vi "dmm_loop_copy_paste_array.vi"(10 "UUT single-ended scan array ref":refnum<vi>, 11 "Copypaste commloop ref":refnum<vi>) -> ()   [LabVIEW 2012]
panel:
  in  "Protocol definition":T1(array[cluster]) {"Variables" items=["Undefined", "Density", "Delta to", "DZDT DeltaT", "Drive mA", "Board Temp", "Mass Flow", "Tube Frequency", "LPO Amp (Filt)", "RPO Amp (Filt)", "LPO Amp (Pk Det)", "RPO Amp (Pk Det)", "Mass Total", "CP Input Volts", "Temp Line", "Drive Gain%", "Flow cal factor", "Status Word 1", "Status Word 2", "Status Word 3", "Status Word 4", "Status Word 5", "Status Word 6"]; "Protocols" items=["None", "MODBUS", "HART", "Fieldbus", "Profibus DP", "Profibus PA"]}
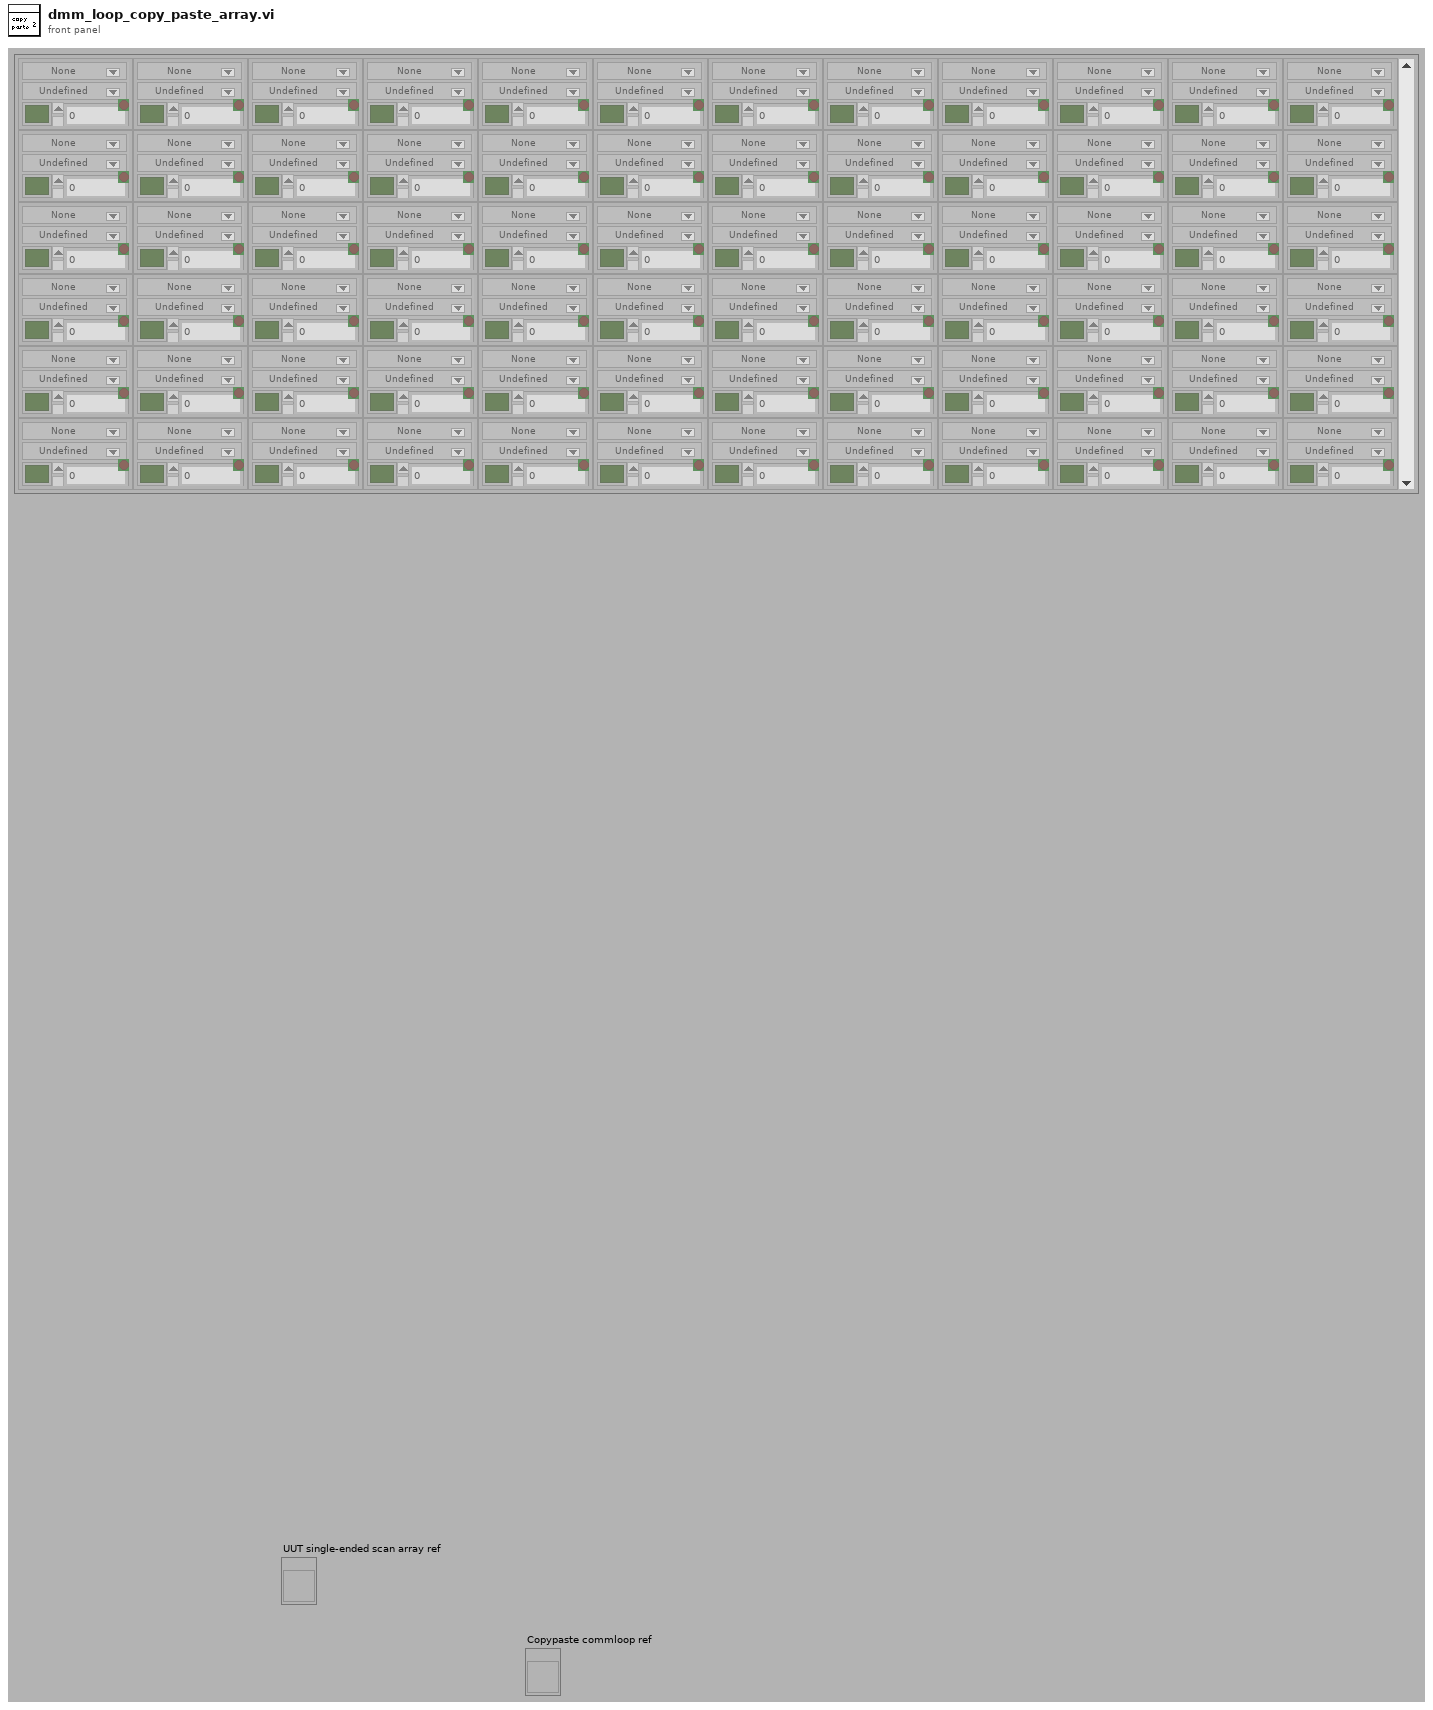
[diagram p1: front panel]
types:
  T1 = cluster{"Protocols":u16, "Variables":u16, "Value":dbl, "Enabled":bool, "Error":bool}[][]
  T2 = cluster{"on?":bool, "Label":string, "measurement type":enum16{"Voltage", "Frequency", "Resistance"}, "Numeric 2":dbl, "current time":timestamp}[][]
  T3 = cluster{"on?":bool, "Label":string, "measurement type":enum16{"Voltage", "Frequency"}, "Numeric 2":dbl, "current time":timestamp}
  T4 = cluster{"on?":bool, "Label":string, "measurement type":enum16{"Voltage", "Frequency", "Resistance"}, "Numeric 2":dbl, "current time":timestamp}[]
  T5 = cluster{"on?":bool, "Label":string, "measurement type":enum16{"Voltage", "Frequency"}, "Numeric 2":dbl, "current time":timestamp}[]
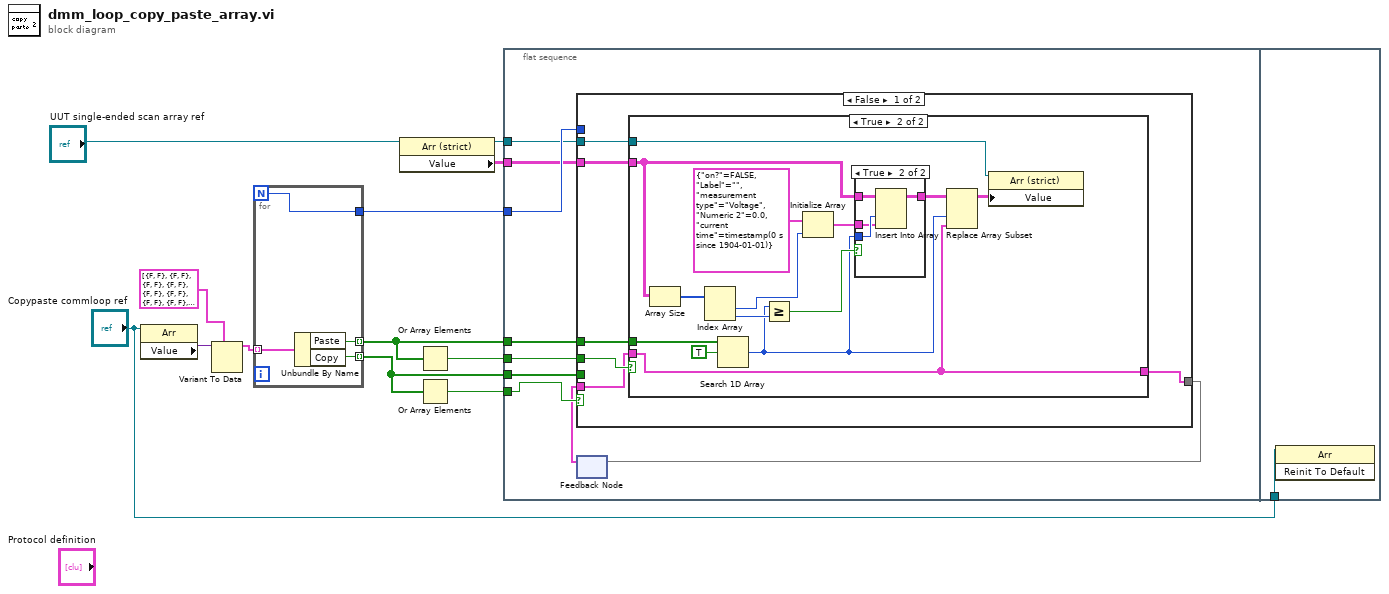
[diagram p0: block diagram]
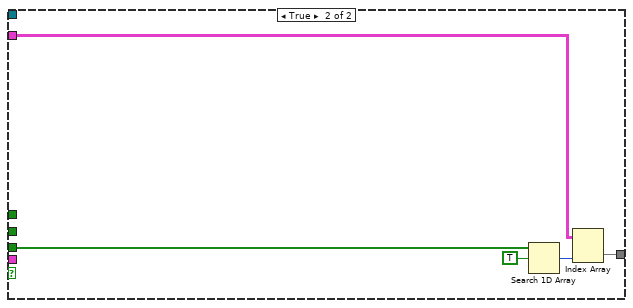
[diagram p4: hidden frame]
diagram:
  n1 = property class="Arr"(reference="Copypaste commloop ref") -> ("Value"=w6:variant)  [unwired: 1 in, 2 out]
  n2 = Variant To Data(type=cluster{"Copy":bool, "Paste":bool}[] [{"Copy"=FALSE, "Paste"=FALSE}, {"Copy"=FALSE, "Paste"=FALSE}, {"Copy"=FALSE, "Paste"=FALSE}, {"Copy"=FALSE, "Paste"=FALSE}, {"Copy"=FALSE, "Paste"=FALSE}, {"Copy"=FALSE, "Paste"=FALSE}, {"Copy"=FALSE, "Paste"=FALSE}, {"Copy"=FALSE, "Paste"=FALSE}, {"Copy"=FALSE, "Paste"=FALSE}, {"Copy"=FALSE, "Paste"=FALSE}, {"Copy"=FALSE, "Paste"=FALSE}, {"Copy"=FALSE, "Paste"=FALSE}] ("Copypaste commloop"), Variant=w6) -> (data=w4:cluster{"Copy":bool, "Paste":bool}[])  [unwired: 1 in, 1 out]
  n3 = for {
    N -> [w13]
    tunnel: w4 -> [w16] mode=indexing
    tunnel: [w15] -> w8 mode=indexing
    tunnel: [w14] -> w10 mode=indexing
    tunnel: [w13] -> w9
    n4 = Unbundle By Name(w16) -> ("Paste"=w15:bool, "Copy"=w14:bool)
  }
  n5 = property class="Arr (strict)"(reference="UUT single-ended scan array ref") -> (reference out=w2:refnum<vi>, "Value"=w3:T2)  [unwired: 1 in, 1 out]
  n6 = Or Array Elements(Boolean array=w8) -> (logical OR=w11:bool)
  n7 = Or Array Elements(Boolean array=w10) -> (logical OR=w12:bool)
  n8 = flat-sequence {
    tunnel: w12 -> [w25]
    tunnel: w11 -> [w24]
    tunnel: w10 -> [w23]
    tunnel: w9 -> [w22]
    tunnel: w8 -> [w19]
    tunnel: w3 -> [w18]
    tunnel: w2 -> [w17]
    tunnel: "Copypaste commloop ref" -> [w57]
    frame #0 {
      n9 = feedback #1() -> (w20:T4)  [unwired: 1 in]
      n10 = case shown="False" w25 {
        tunnel: w24 -> [w31 _]
        tunnel: w23 -> [_ w56]
        tunnel: w22 -> [_ _]
        tunnel: [w28 w55] -> w21
        tunnel: w20 -> [w30 _]
        tunnel: w19 -> [w29 _]
        tunnel: w18 -> [w27 w52]
        tunnel: w17 -> [w26 _]
        frame False {
          n11 = case shown="True" w31 {
            tunnel: w30 -> [w32 w41]
            tunnel: w29 -> [_ w45]
            tunnel: [w32 w41] -> w28
            tunnel: w27 -> [_ w40]
            tunnel: w26 -> [_ w38]
            frame False {
            }
            frame True {
              n12 = Array Size(array=w40) -> (size(s)=w44:i32[])
              n13 = Index Array(array=w44) -> (element #1=w35:i32, element #2=w37:i32)  [unwired: 2 in]
              n14 = Search 1D Array(1D array=w45, element=TRUE) -> (index of element=w34:i32)  [unwired: 1 in]
              n15 = Greater Or Equal?(x=w34, y=w37) -> (x >= y?=w43:bool)
              n16 = Initialize Array(T3 {"on?"=FALSE, "Label"="", "measurement type"=enum."Voltage", "Numeric 2"=0.0, "current time"=timestamp(0 s since 1904-01-01)} ("Cluster 2"), w35) -> (w36:T5)
              n17 = case shown="True" w43 {
                tunnel: w40 -> [w47 w51]
                tunnel: [w47 w50] -> w42
                tunnel: w36 -> [_ w48]
                tunnel: w34 -> [_ w49]
                frame False {
                }
                frame True {
                  n18 = Insert Into Array(array=w51, index (col)=w49, new element=w48) -> (w50:T2)  [unwired: 1 in]
                }
              }
              n19 = Replace Array Subset(array=w42, new element=w41, index (col)=w34) -> (w39:T2)  [unwired: 1 in]
              n20 = property class="Arr (strict)"(reference=w38, "Value"=w39) -> ()  [unwired: 1 in, 2 out]
            }
          }
        }
        frame True {
          n21 = Search 1D Array(1D array=w56, element=TRUE) -> (index of element=w53:i32)  [unwired: 1 in]
          n22 = Index Array(array=w52, index (col)=w53) -> (element=w55:T4)  [unwired: 1 in]
        }
      }
      n23 = feedback-in #1(w21) -> ()
    }
    frame #1 {
      n24 = invoke class="Arr" method="Reinit To Default"(reference=w57) -> ()  [unwired: 2 in, 3 out]
    }
  }
